vi "Main.vi"(11 "Module Admin":refnum<class "Delacor_lib_QMH_Module Admin.lvclass">) -> ()   [LabVIEW 2020, in "UI.lvlib"]
doc: "This template is based off of the Queued Message Handler design pattern and the Queued Message Handler project template that ships with LabVIEW.\n\nThe main difference is that the queue is private to this module and communication between modules is performed via Broadcast and Request events.\n\nRequest events are wrapped in public API methods and are handled in the Event Handling Loop (EHL) of this VI. Any module can register for Broadcast events sent by this module. The EHL generates messages based on user interface actions.\n\nThe Message Handling Loop (MHL) processes messages generated by the EHL, or by other messages. The messages are string values, so new messages can be added easily to the Message Cases case structure in the MHL. Each message cluster can also provide an optional value for Message Data, which is a variant that can be converted to whatever message-specific data is required.\n_____\nBased on Delacor QMH Project Template 5.0.0.82."
uses:
  UI.lvlib
  <vilib>/Delacor/Delacor QMH/Libraries/Module Admin_class/Delacor_lib_QMH_Module Admin.lvclass
  Module Data--cluster.ctl
  Stop Argument--cluster.ctl
  <vilib>/Delacor/Delacor QMH/Libraries/Message Queue_class/Delacor_lib_QMH_Message Queue.lvclass/Delacor_lib_QMH_Message Queue.ctl
  <vilib>/Delacor/Delacor QMH/Libraries/Module Admin_class/Delacor_lib_QMH_Module Admin.lvclass/Delacor_lib_QMH_Module Admin.ctl
  <vilib>/Delacor/Delacor QMH/Libraries/Message Queue_class/Delacor_lib_QMH_Enqueue Message (Single).vi
  <vilib>/Delacor/Delacor QMH/Libraries/Module Admin_class/Delacor_lib_QMH_Get External Launch.vi
  <vilib>/Utility/error.llb/Error Cluster From Error Code.vi
  <vilib>/ErrorRing/Error Ring.xnode
  <vilib>/Delacor/Delacor QMH/Libraries/Message Queue_class/Delacor_lib_QMH_Message Queue.lvclass
  Acquisition/Acquisition.lvlib
panel:
  in  "Delay":i32
  in  "Stop":bool
  in  "Start":bool
  out "error out":errorcluster
  out "Status":string
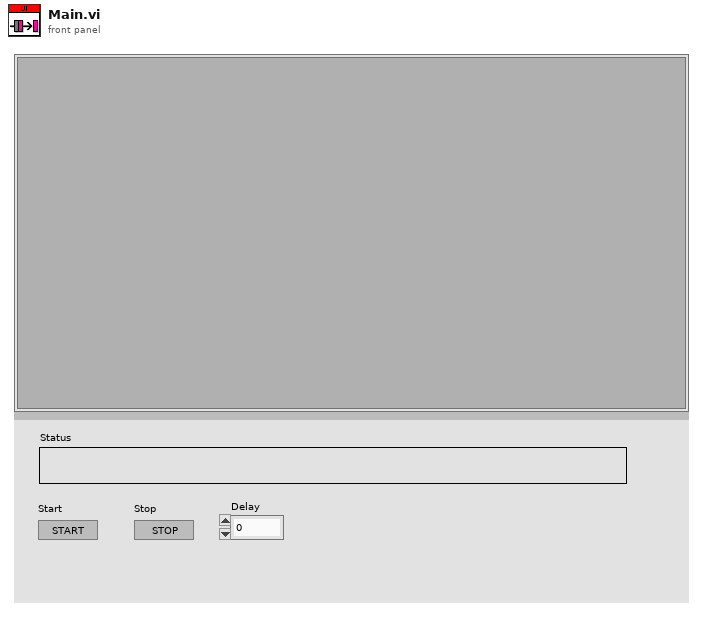
[diagram p1: front panel]
types:
  T1 = typedef "UI.lvlib/Request Events--cluster.ctl" = cluster{"Stop Module":refnum<user-event>, "Show Panel":refnum<user-event>, "Hide Panel":refnum<user-event>, "Get Module Execution Status":refnum<user-event>, "Show Diagram":refnum<user-event>}
  T2 = typedef "Acquisition.lvlib/Broadcast Events--cluster.ctl" = cluster{"Module Did Init":refnum<user-event>, "Status Updated":refnum<user-event>, "Error Reported":refnum<user-event>, "Module Did Stop":refnum<user-event>, "Update Module Execution Status":refnum<user-event>}
  T3 = typedef "UI.lvlib/Module Data--cluster.ctl" = cluster{"Status":string}
  T4 = enum32{"invalid lock state", "Not Locked", "Locked (No Password)", "Password-protected"}
  T5 = typedef "UI.lvlib/Stop Argument--cluster.ctl" = cluster{"Origin":string, "Exit via Stop Module Req?":bool, "Wait for Module to stop?":bool}
  T6 = enum32{"Invalid", "Standard", "Closed", "Hidden", "Minimized", "Maximized"}
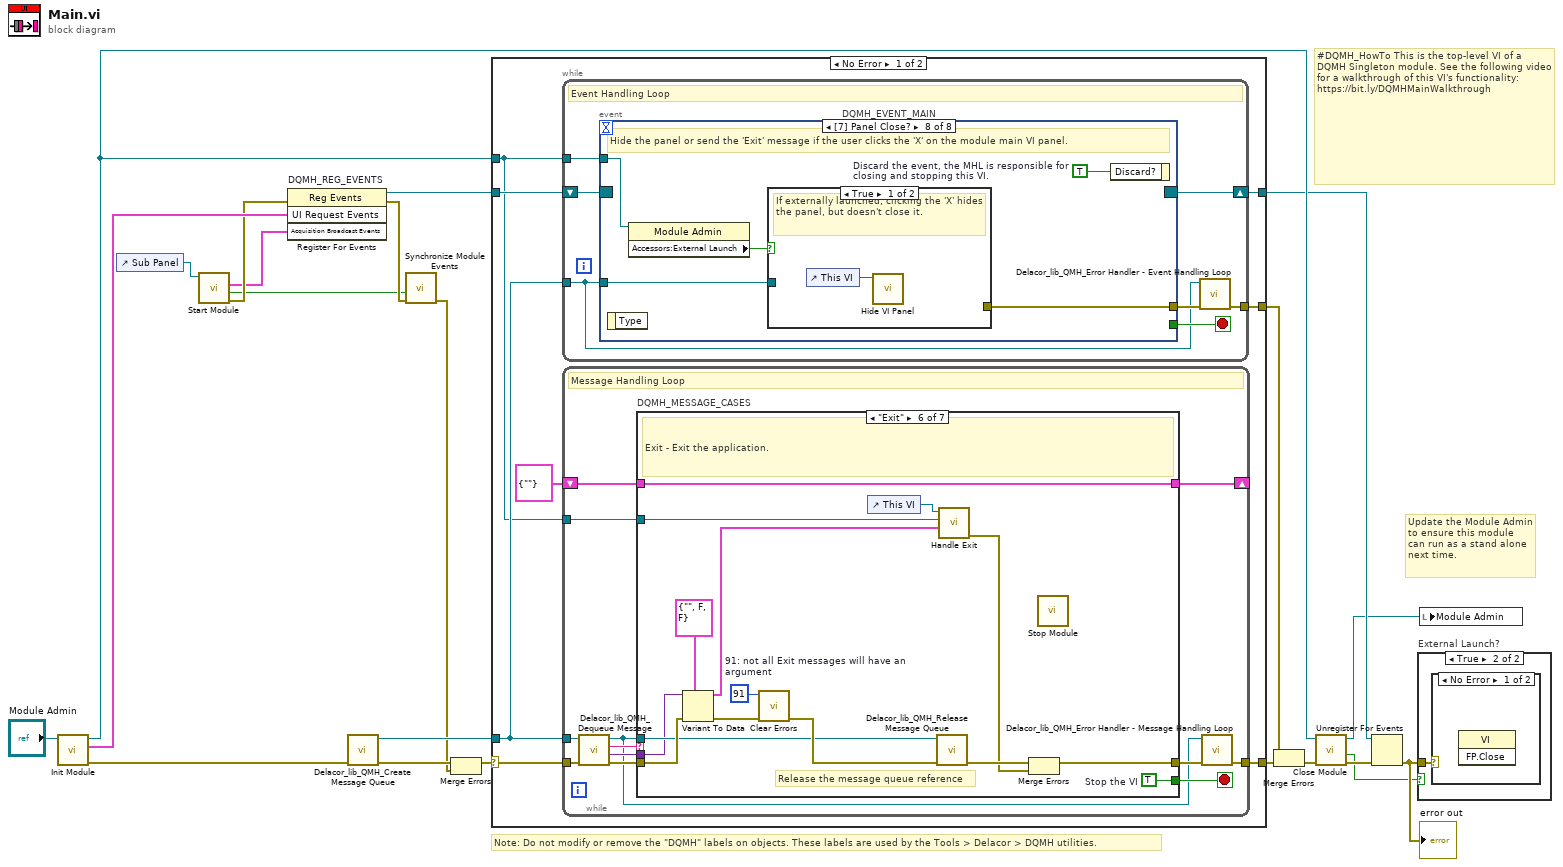
[diagram p0: block diagram]
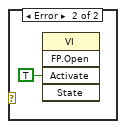
[diagram p3: hidden frame]
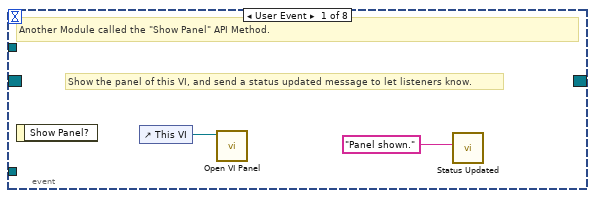
[diagram p4: hidden frame]
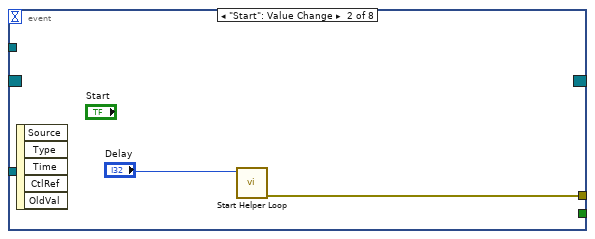
[diagram p5: hidden frame]
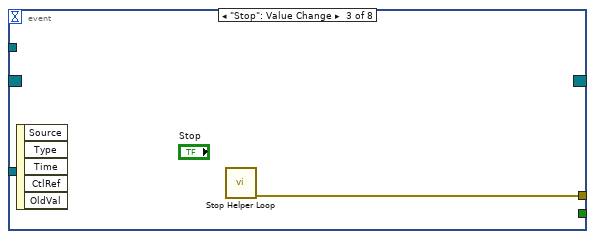
[diagram p6: hidden frame]
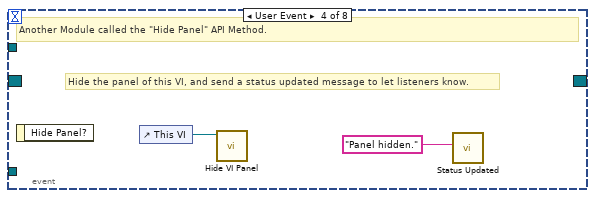
[diagram p7: hidden frame]
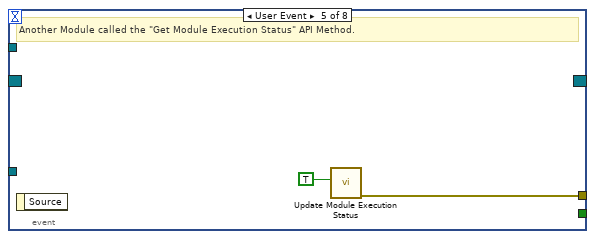
[diagram p8: hidden frame]
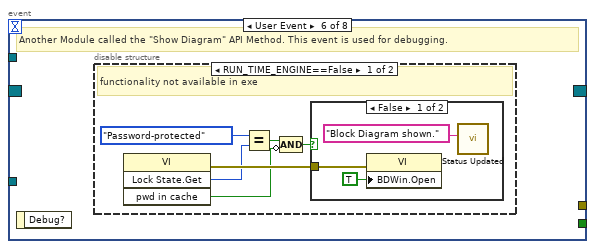
[diagram p9: hidden frame]
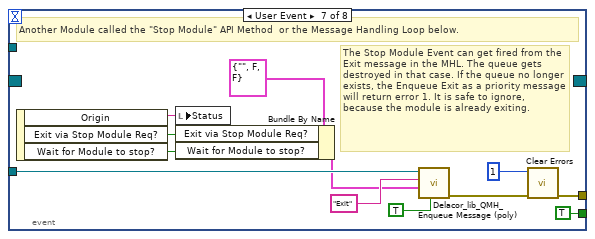
[diagram p12: hidden frame]
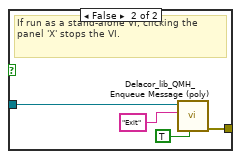
[diagram p13: hidden frame]
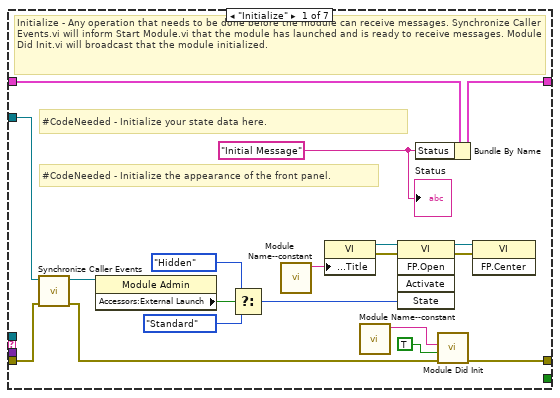
[diagram p14: hidden frame]
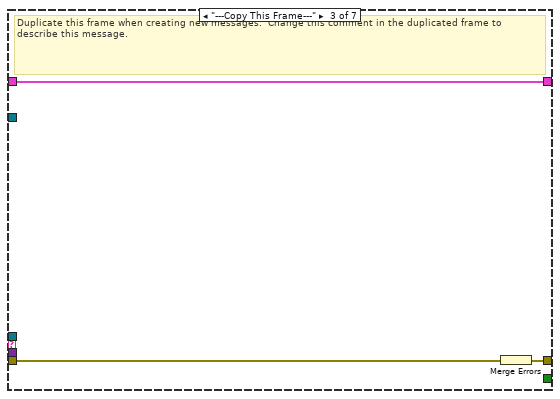
[diagram p16: hidden frame]
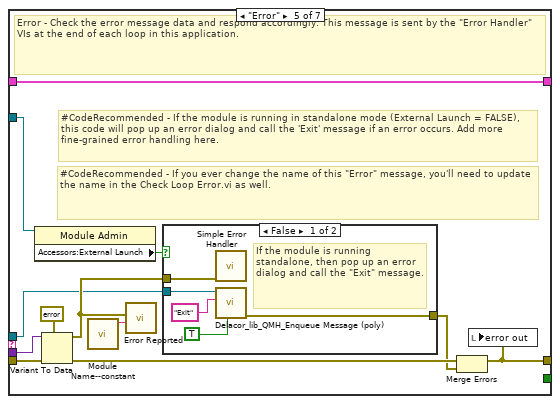
[diagram p18: hidden frame]
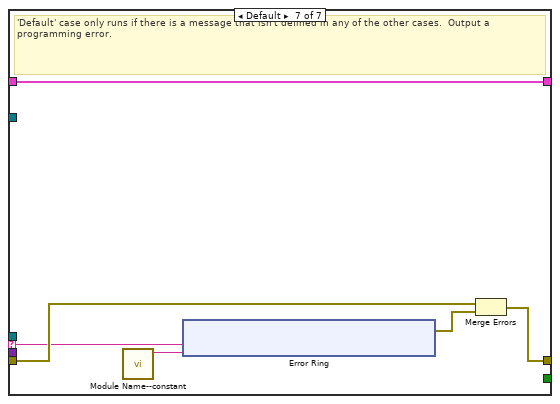
[diagram p20: hidden frame]
diagram:
  # "#DQMH_HowTo This is the top-level VI of a DQMH Singleton module. See the following video for a walkthrough of this VI's functionality: https://bit.ly/DQMHMainWalkthrough"
  # "Note: Do not modify or remove the \"DQMH\" labels on objects. These labels are used by the Tools > Delacor > DQMH utilities."
  # "Update the Module Admin to ensure this module can run as a stand alone next time."
  n1 = call "Init Module.vi"("Singleton Module Admin in"="Module Admin") -> ("error out"=w21:errorcluster, "UI Request Events"=w11:T1, "Singleton Module Admin out"=w14:refnum<class "Delacor_lib_QMH_Module Admin.lvclass">)  [unwired: 8 in]
  n2 = control-ref of="Sub Panel"() -> (w6:refnum<vi>)
  n3 = call "Start Module.vi"("Sub Panel"=w6) -> ("error out"=w5:errorcluster, "Wait for Event Sync?"=w1:bool, "Acquisition Broadcast Events"=w4:T2)  [unwired: 7 in, 1 out]
  n4 = register-events "DQMH_REG_EVENTS"(error in=w5, w11, w4) -> (reference out=w12:refnum<event-registration>, error out=w3:errorcluster)  [unwired: 1 in]
  n5 = call <vilib>:"Delacor_lib_QMH_Create Message Queue.vi"("error in (no error)"=w21) -> ("error out"=w16:errorcluster, "Message Queue"=w10:refnum<class "Delacor_lib_QMH_Message Queue.lvclass">)  [unwired: 9 in]
  n6 = call "Synchronize Module Events.vi"("error in (no error)"=w3, "Wait for Event Sync?"=w1) -> ("error out"=w2:errorcluster)  [unwired: 9 in]
  n7 = Merge Errors(w16, w2) -> (w15:errorcluster)
  n8 = case shown="No Error" w15 {
    selector: w15 -> [w28 w164]
    tunnel: [w30 w163] -> w22
    tunnel: [w27 w169] -> w13
    tunnel: w12 -> [w25 w169]
    tunnel: w10 -> [w24 w162]
    tunnel: [w29 _] -> w19
    tunnel: w14 -> [w23 w165]
    frame No Error {
      n9 = while {
        tunnel: w24 -> [w31]
        shift-right: [w34] -> w27
        shift-left: w25 -> [w35]
        tunnel: [w36] -> w29
        tunnel: w23 -> [w32]
        stop <- w33 stop-if-true
        # "Event Handling Loop"
        n10 = event "DQMH_EVENT_MAIN" shown="[7] Panel Close?" {
          selector: w35 -> [_ _ _ _ _ _ _ _]
          dyn-events: [_ _ _ _ _ _ _ _] -> w34
          timeout: _ -> [_ _ _ _ _ _ _ _]
          tunnel: [_ _ _ _ _ _ TRUE ("Discard?") _] -> w33
          tunnel: w31 -> [_ _ _ _ _ _ w63 w70]
          tunnel: [_ w41 w42 _ w46 _ w66 w72] -> w37
          tunnel: w32 -> [_ _ _ _ _ _ _ w69]
          event User Event {
            # "Show the panel of this VI, and send a status updated message to let listeners know."
            # "Another Module called the \"Show Panel\" API Method."
            n11 = event-data() -> ()  [unwired: 1 in, 1 out]
            n12 = control-ref of="This VI"() -> (w39:refnum<vi>)
            n13 = call "Open VI Panel.vi"("VI"=w39) -> ()  [unwired: 10 in, 1 out]
            n14 = call "Status Updated.vi"("Status"="Panel shown." ("format string")) -> ()  [unwired: 10 in, 1 out]
          }
          event "Start": Value Change {
            n15 = event-data() -> ()  [unwired: 1 in, 5 out]
            n16 = call "Start Helper Loop.vi"("DELAY Timeout"="Delay") -> ("error out"=w41:errorcluster)  [unwired: 10 in]
          }
          event "Stop": Value Change {
            n17 = event-data() -> ()  [unwired: 1 in, 5 out]
            n18 = call "Stop Helper Loop.vi"() -> ("error out"=w42:errorcluster)  [unwired: 11 in]
          }
          event User Event {
            # "Hide the panel of this VI, and send a status updated message to let listeners know."
            # "Another Module called the \"Hide Panel\" API Method."
            n19 = event-data() -> ()  [unwired: 1 in, 1 out]
            n20 = control-ref of="This VI"() -> (w44:refnum<vi>)
            n21 = call "Hide VI Panel.vi"("VI"=w44) -> ()  [unwired: 10 in, 1 out]
            n22 = call "Status Updated.vi"("Status"="Panel hidden." ("format string")) -> ()  [unwired: 10 in, 1 out]
          }
          event User Event {
            # "Another Module called the \"Get Module Execution Status\" API Method."
            n23 = event-data() -> ()  [unwired: 1 in, 1 out]
            n24 = call "Update Module Execution Status.vi"("Running?"=TRUE) -> ("error out"=w46:errorcluster)  [unwired: 10 in]
          }
          event User Event {
            # "Another Module called the \"Show Diagram\" API Method. This event is used for debugging."
            n25 = event-data() -> ()  [unwired: 1 in, 1 out]
            n26 = disable-structure shown="RUN_TIME_ENGINE==False" {
              frame condition #0 (active) {
                # "functionality not available in exe"
                n27 = invoke class="VI" method="Lock State.Get"() -> (error out=w52:errorcluster, "Get Lock State"=w51:T4, "pwd in cache"=w48:bool)  [unwired: 4 in, 1 out]
                n28 = Equal?(x=T4."Password-protected", y=w51) -> (x = y?=w49:bool)
                n29 = Compound Arithmetic op=AND(w49, invert w48) -> (w47:bool)
                n30 = case shown="False" w47 {
                  tunnel: w52 -> [w55 _]
                  frame False {
                    n31 = property class="VI"(error in=w55, "BDWin.Open"=TRUE ("Block Diagram Window:Open")) -> ()  [unwired: 1 in, 2 out]
                    n32 = call "Status Updated.vi"("Status"="Block Diagram shown." ("format string")) -> ()  [unwired: 10 in, 1 out]
                  }
                  frame True {
                    # "Password-protected VI, and the password is not in the cache. Do not show the diagram."
                  }
                }
              }
              frame condition #1 {
              }
            }
          }
          event User Event {
            # "The Stop Module Event can get fired from the Exit message in the MHL. The queue gets destroyed in that case. If the queue no longer exists, the Enqueue Exit as a priority message will return error 1. It is safe to ignore, because the module is already exiting."
            # "Another Module called the \"Stop Module\" API Method  or the Message Handling Loop below."
            n33 = event-data() -> ("Origin"=w62:string, "Exit via Stop Module Req?"=w58:bool, "Wait for Module to stop?"=w57:bool)  [unwired: 1 in]
            n34 = local write "Status"(w62) -> ()
            n35 = Bundle By Name(cluster=T5 {"Origin"="", "Exit via Stop Module Req?"=FALSE, "Wait for Module to stop?"=FALSE} ("Stop Argument"), "Exit via Stop Module Req?"=w58, "Wait for Module to stop?"=w57) -> (w56:T5)
            n36 = call-poly <vilib>:"Delacor_lib_QMH_Enqueue Message (poly).vi"("Priority Message? (F)"=TRUE, "Message Data"=w56, "Message"="Exit", "Message Queue in"=w63) -> ("error out"=w67:errorcluster)  [unwired: 6 in, 1 out]
            n37 = call <vilib>:"Clear Errors.vi"("error in (no error)"=w67, "specific error code to clear (0: all)"=1) -> ("error out"=w66:errorcluster)  [unwired: 4 in, 1 out]
          }
          event Panel Close? {
            w71 = TRUE  # Discard the event, the MHL is responsible for closing and stopping this VI.
            # "Hide the panel or send the 'Exit' message if the user clicks the 'X' on the module main VI panel."
            n38 = event-data() -> ()  [unwired: 1 in, 1 out]
            n39 = property class="Module Admin"(reference=w69) -> ("Accessors:External Launch"=w68:bool)  [unwired: 1 in, 2 out]
            n40 = case shown="True" w68 {
              tunnel: w70 -> [_ w76]
              tunnel: [_ w77] -> w72
              frame True {
                # "If externally launched, clicking the 'X' hides the panel, but doesn't close it."
                n41 = control-ref of="This VI"() -> (w73:refnum<vi>)
                n42 = call "Hide VI Panel.vi"("VI"=w73) -> ()  [unwired: 10 in, 1 out]
              }
              frame False {
                # "If run as a stand-alone VI, clicking the panel 'X' stops the VI."
                n43 = call-poly <vilib>:"Delacor_lib_QMH_Enqueue Message (poly).vi"("Priority Message? (F)"=TRUE, "Message"="Exit", "Message Queue in"=w76) -> ("error out"=w77:errorcluster)  [unwired: 7 in, 1 out]
              }
            }
            n44 = event-data("Discard?"=w71) -> ()  [unwired: 1 in, 1 out]
          }
        }
        n45 = call-dynamic "Delacor_lib_QMH_Error Handler - Event Handling Loop.vi"("error in (no error)"=w37, "Message Queue in"=w31) -> ("dup error in"=w36:errorcluster)  [unwired: 8 in, 1 out]
      }
      n46 = while {
        tunnel: w24 -> [w80]
        shift-right: [w84] -> _
        shift-left: T3 {"Status"=""} ("Data Cluster") -> [w85]
        tunnel: w28 -> [w88]
        tunnel: [w86] -> w30
        tunnel: w23 -> [w78]
        stop <- w83 stop-if-true
        # "Message Handling Loop"
        n47 = call-dynamic "Delacor_lib_QMH_Dequeue Message.vi"("error in (no error)"=w88, "Message Queue in"=w80) -> ("error out"=w87:errorcluster, "Message Data"=w81:variant, "Message"=w82:string, "Message Queue out"=w79:refnum<class "Delacor_lib_QMH_Message Queue.lvclass">)  [unwired: 6 in]
        n48 = case "DQMH_MESSAGE_CASES" shown="\"Exit\"" w82 {
          selector: w82 -> [_ _ _ _ _ _ w149]
          tunnel: w79 -> [_ _ _ _ w119 w141 _]
          tunnel: w87 -> [w106 w110 w113 w115 w126 w147 w151]
          tunnel: [w104 w110 w112 w115 w122 w144 w152] -> w89
          tunnel: w85 -> [w95 w109 w111 w114 w121 w140 w150]
          tunnel: [w94 w109 w111 w114 w121 w140 w150] -> w84
          tunnel: [_ _ _ _ _ w139 _] -> w83
          tunnel: w81 -> [_ _ _ _ w120 w138 _]
          tunnel: w78 -> [w96 _ _ _ w118 w133 _]
          frame "Initialize" {
            w90 = "Initial Message" ("Initial Message")
            # "#CodeNeeded - Initialize the appearance of the front panel."
            # "#CodeNeeded - Initialize your state data here."
            # "Initialize - Any operation that needs to be done before the module can receive messages. Synchronize Caller Events.vi will inform Start Module.vi that the module has launched and is ready to receive messages. Module Did Init.vi will broadcast that the module initialized."
            n49 = call "Synchronize Caller Events.vi"("error in (no error)"=w106, "Singleton Module Admin in"=w96) -> ("error out"=w105:errorcluster, "Singleton Module Admin out"=w91:refnum<class "Delacor_lib_QMH_Module Admin.lvclass">)  [unwired: 8 in]
            n50 = property class="Module Admin"(reference=w91) -> ("Accessors:External Launch"=w100:bool)  [unwired: 1 in, 2 out]
            n51 = Select(t=T6."Hidden" ("State"), s=w100, f=T6."Standard" ("State")) -> (s? t:f=w97:T6)
            n52 = call "Module Name--constant.vi"() -> ("Module Name"=w103:string)  [unwired: 11 in]
            n53 = property class="VI"("Front Panel.Title"=w103) -> (reference out=w102:refnum<vi>, error out=w108:errorcluster)  [unwired: 2 in]
            n54 = call "Module Name--constant.vi"() -> ("Module Name"=w92:string)  [unwired: 11 in]
            n55 = invoke class="VI" method="FP.Open"(reference=w102, error in=w108, "State"=w97) -> (reference out=w101:refnum<vi>, error out=w107:errorcluster)  [unwired: 2 in, 3 out]
            n56 = Bundle By Name(cluster=w95, "Status"=w90) -> (w94:T3)
            n57 = call "Module Did Init.vi"("error in (no error)"=w105, "Initialized?"=TRUE, "Origin"=w92) -> ("error out"=w104:errorcluster)  [unwired: 8 in]
            n58 = invoke class="VI" method="FP.Center"(reference=w101, error in=w107) -> ()  [unwired: 1 in, 3 out]
            "Status" <- w90
          }
          frame "--- Module Specific ---" {
            # "Separator -- The following cases handle messages specific to this Module."
          }
          frame "---Copy This Frame---" {
            # "Duplicate this frame when creating new messages.  Change this comment in the duplicated frame to describe this message."
            n59 = Merge Errors(w113) -> (w112:errorcluster)
          }
          frame "--- Exit and Error Handling---" {
            # "Separator - The following cases handle errors and exit messages."
          }
          frame "Error" {
            # "#CodeRecommended - If you ever change the name of this \"Error\" message, you'll need to update the name in the Check Loop Error.vi as well."
            # "#CodeRecommended - If the module is running in standalone mode (External Launch = FALSE), this code will pop up an error dialog and call the 'Exit' message if an error occurs. Add more fine-grained error handling here."
            # "Error - Check the error message data and respond accordingly. This message is sent by the \"Error Handler\" VIs at the end of each loop in this application."
            n60 = property class="Module Admin"(reference=w118) -> ("Accessors:External Launch"=w117:bool)  [unwired: 1 in, 2 out]
            n61 = Variant To Data(error in=w126, type=errorcluster {"status"=FALSE, "code"=0, "source"=""} ("error constant"), Variant=w120) -> (data=w127:errorcluster, error out=w124:errorcluster)
            n62 = call "Module Name--constant.vi"() -> ("Module Name"=w116:string)  [unwired: 11 in]
            n63 = call "Error Reported.vi"("Additional Information"=w116, "Error"=w127) -> ()  [unwired: 9 in, 1 out]
            n64 = case shown="False" w117 {
              tunnel: [w132 _] -> w123
              tunnel: w119 -> [w130 _]
              tunnel: w127 -> [w131 _]
              frame False {
                # "If the module is running standalone, then pop up an error dialog and call the \"Exit\" message."
                n65 = call <vilib>:"Simple Error Handler.vi"("error in (no error)"=w131) -> ()  [unwired: 4 in, 5 out]
                n66 = call-poly <vilib>:"Delacor_lib_QMH_Enqueue Message (poly).vi"("Priority Message? (F)"=TRUE, "Message"="Exit", "Message Queue in"=w130) -> ("error out"=w132:errorcluster)  [unwired: 7 in, 1 out]
              }
              frame True {
                # "If the module was launched externally, calling the Error Reported broadcast VI is the only action performed by the \"Error\" message. The module's caller can then process the error appropriately."
              }
            }
            n67 = Merge Errors(w124, w123) -> (w122:errorcluster)
            n68 = local write "error out"(w122) -> ()
          }
          frame "Exit" {
            w137 = 91  # 91: not all Exit messages will have an argument
            w139 = TRUE  # Stop the VI
            # "Release the message queue reference"
            # "Exit - Exit the application."
            n69 = Variant To Data(error in=w147, type=T5 {"Origin"="", "Exit via Stop Module Req?"=FALSE, "Wait for Module to stop?"=FALSE} ("Stop Argument"), Variant=w138) -> (data=w135:T5, error out=w143:errorcluster)
            n70 = call <vilib>:"Clear Errors.vi"("error in (no error)"=w143, "specific error code to clear (0: all)"=w137) -> ("error out"=w146:errorcluster)  [unwired: 4 in, 1 out]
            n71 = control-ref of="This VI"() -> (w134:refnum<vi>)
            n72 = call-dynamic "Delacor_lib_QMH_Release Message Queue.vi"("error in (no error)"=w146, "Message Queue"=w141) -> ("error out"=w145:errorcluster)  [unwired: 9 in]
            n73 = call "Handle Exit.vi"("Stop Argument"=w135, "Admin in"=w133, "VI reference"=w134) -> ("error out"=w142:errorcluster)  [unwired: 7 in, 1 out]
            n74 = Merge Errors(w145, w142) -> (w144:errorcluster)
            n75 = call "Stop Module.vi"() -> ()  [unwired: 11 in, 1 out]
          }
          frame Default {
            # "'Default' case only runs if there is a message that isn't defined in any of the other cases.  Output a programming error."
            n76 = call "Module Name--constant.vi"() -> ("Module Name"=w148:string)  [unwired: 11 in]
            n77 = xnode "Error Ring"("parameter 0"=w149, "parameter 1"=w148) -> ("error out"=w153:errorcluster)
            n78 = Merge Errors(w151, w153) -> (w152:errorcluster)
          }
        }
        n79 = call-dynamic "Delacor_lib_QMH_Error Handler - Message Handling Loop.vi"("error in (no error)"=w89, "Message Queue in"=w79) -> ("dup error in"=w86:errorcluster)  [unwired: 8 in, 1 out]
      }
    }
    frame Error {
      # "Synchronize Caller Events.vi will inform Start Module.vi that the module has launched and will let the code calling Start Module.vi register for broadcasts and would permit the caller receive the broadcast that an error occurred at launch time."
      n80 = call-dynamic "Delacor_lib_QMH_Release Message Queue.vi"("error in (no error)"=w164, "Message Queue"=w162) -> ("error out"=w163:errorcluster)  [unwired: 9 in]
      n81 = call "Synchronize Caller Events.vi"("Singleton Module Admin in"=w165) -> ("error out"=w170:errorcluster)  [unwired: 9 in, 1 out]
      n82 = call "Module Name--constant.vi"() -> ("Module Name"=w168:string)  [unwired: 11 in]
      n83 = Format Into String(format string="An error occurred during initialization. %s is no longer running.", w168) -> (resulting string=w166:string)  [unwired: 2 in, 1 out]
      n84 = Merge Errors(w163, w170) -> (w171:errorcluster)
      n85 = call "Error Reported.vi"("Additional Information"=w166, "Error"=w171) -> ()  [unwired: 9 in, 1 out]
    }
  }
  n86 = Merge Errors(w19, w22) -> (w18:errorcluster)
  n87 = call "Close Module.vi"("error in (no error)"=w18, "Module Admin in"=w14) -> ("error out"=w20:errorcluster, "External Launch"=w7:bool, "Module Admin out"=w8:refnum<class "Delacor_lib_QMH_Module Admin.lvclass">)  [unwired: 7 in]
  n88 = Unregister For Events(event registration refnum=w13, error in=w20) -> (error out=w17:errorcluster)
  "error out" <- w17
  n89 = case "External Launch?" shown="True" w7 {
    tunnel: w17 -> [_ w172]
    frame False {
    }
    frame True {
      n90 = case shown="No Error" w172 {
        frame No Error {
          n91 = invoke class="VI" method="FP.Close"() -> ()  [unwired: 3 in, 3 out]
        }
        frame Error {
          n92 = invoke class="VI" method="FP.Open"("Activate"=TRUE ("Activate?")) -> ()  [unwired: 4 in, 5 out]
        }
      }
    }
  }
  n93 = local write "Module Admin"(w8) -> ()
